vi "setSlitPosition.vi"(8 "error in (no error)":errorcluster, 9 "Monochromator in":refnum<class "Monochromator.lvclass">, 10 "position":T1, 11 "ReadySate in":refnum<class "ReadySate.lvclass">) -> (0 "error out":errorcluster, 1 "Monochromator out":refnum<class "Monochromator.lvclass">, 3 "ReadySate out":refnum<class "ReadySate.lvclass">)   [LabVIEW 2016, in "ReadySate.lvclass"]
uses:
  ReadySate.lvclass
  Typedefs/slit.ctl
  Typedefs/SlitType.ctl
  Typedefs/slitPosition.ctl
  Monochromator/Monochromator.lvclass
  Typedefs/SWStatus.ctl
  Typedefs/AckType.ctl
  Monochromator/Monochromator.lvclass/Monochromator.ctl
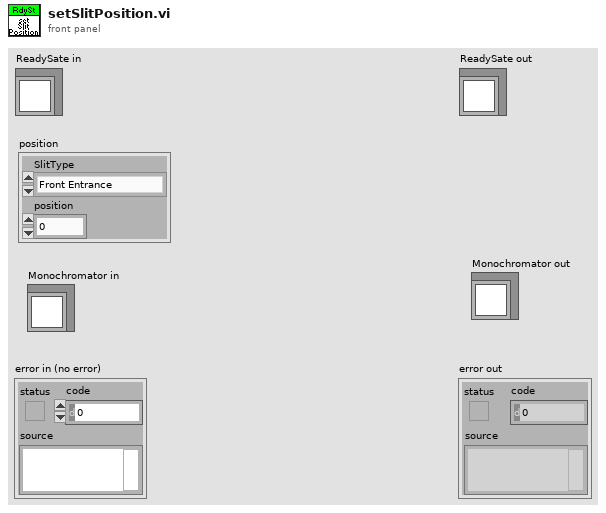
[diagram p1: front panel]
types:
  T1 = typedef "slit.ctl" = cluster{"SlitType":T2, "position":T3}
  T2 = typedef "SlitType.ctl" = enum16{"Front Entrance", "Side Entrance", "Front Exit", "Side Exit", "First Intermediate", "Second Intermediate"}
  T3 = typedef "slitPosition.ctl" = dbl
  T4 = typedef "AckType.ctl" = enum16{"OK", "OutOfRange", "Unknown", "Busy", "Rejected"}
  T5 = typedef "SWStatus.ctl" = enum16{"OfflineState", "ReadyState", "SettingUpState", "FaultState"}
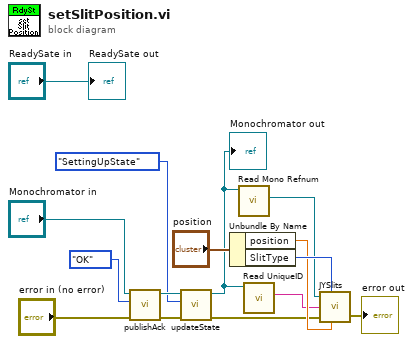
[diagram p0: block diagram]
diagram:
  n1 = call "publishAck.vi"("error in (no error)"="error in (no error)", "Ack"=AckType."OK" ("AckType"), "Monochromator in"="Monochromator in") -> ("error out"=w6:errorcluster, "Monochromator out"=w7:refnum<class "Monochromator.lvclass">)  [unwired: 7 in]
  n2 = call "updateState.vi"("error in (no error)"=w6, "SWStatus"=SWStatus."SettingUpState", "Monochromator in"=w7) -> ("error out"=w3:errorcluster, "Monochromator out"=w1:refnum<class "Monochromator.lvclass">)  [unwired: 7 in]
  "Monochromator out" <- w1
  n3 = Unbundle By Name("position") -> ("position"=w14:T3, "SlitType"=w15:T2)
  n4 = call "Read Mono Refnum.vi"("Monochromator in"=w1) -> ("Mono Refnum"=w10:refnum<k7>)  [unwired: 8 in, 2 out]
  n5 = call "Read UniqueID.vi"("Monochromator in"=w1) -> ("UniqueID"=w9:string)  [unwired: 8 in, 2 out]
  n6 = call "JYSlits.vi"("JYMONOLib.IJYMonoReqd"=w10, "Slit"=w15, "UniqueID"=w9, "error in (no error)"=w3, "Slit Width"=w14) -> ("error out"=→"error out":errorcluster)  [unwired: 1 out]
  "ReadySate out" <- "ReadySate in"
